vi "Read Waveform.vi"(8 "error in (no error)":errorcluster {"code" format="%.0x"}, 10 "Channel":string(combo)="Channel 1", 11 "VISA Resource Name":refnum<visa-resource-name>) -> (0 "error out":errorcluster {"code" format="%.0x"}, 1 "x increment":dbl caption="x Increment" format="%^.2e", 2 "initial x":dbl caption="Initial x" format="%^.2e", 3 "VISA Resource Name Out":refnum<visa-resource-name>, 4 "waveform array":dbl[](array[numeric]) caption="Waveform Array" format="%.2f", 5 "actual points":u32 caption="Actual Points")   [LabVIEW 2015, in "Agilent 546XX Series.lvlib"]
doc: "This VI initiates an acquisition on the channels that you enable with the ag546xx Configure Channel VI. It then waits for the acquisition to complete, and returns the waveform for the channel you specify. You call the ag546xx Fetch Waveform VI to obtain the waveforms for each of the remaining enabled channels without initiating another acquisition.\n\nNotes:\n\n(1) After this VI executes, each element in the Waveform Array is either a voltage or a value indicating that the oscilloscope could not sample a voltage."
uses:
  Agilent 546XX Series.lvlib
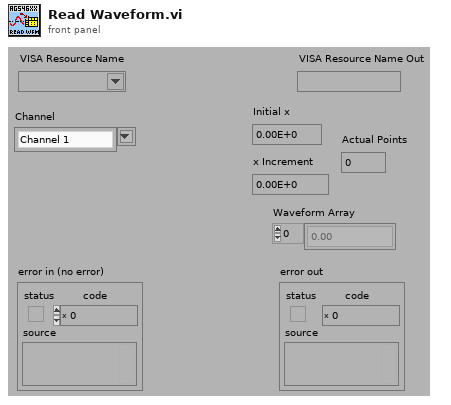
[diagram p1: front panel]
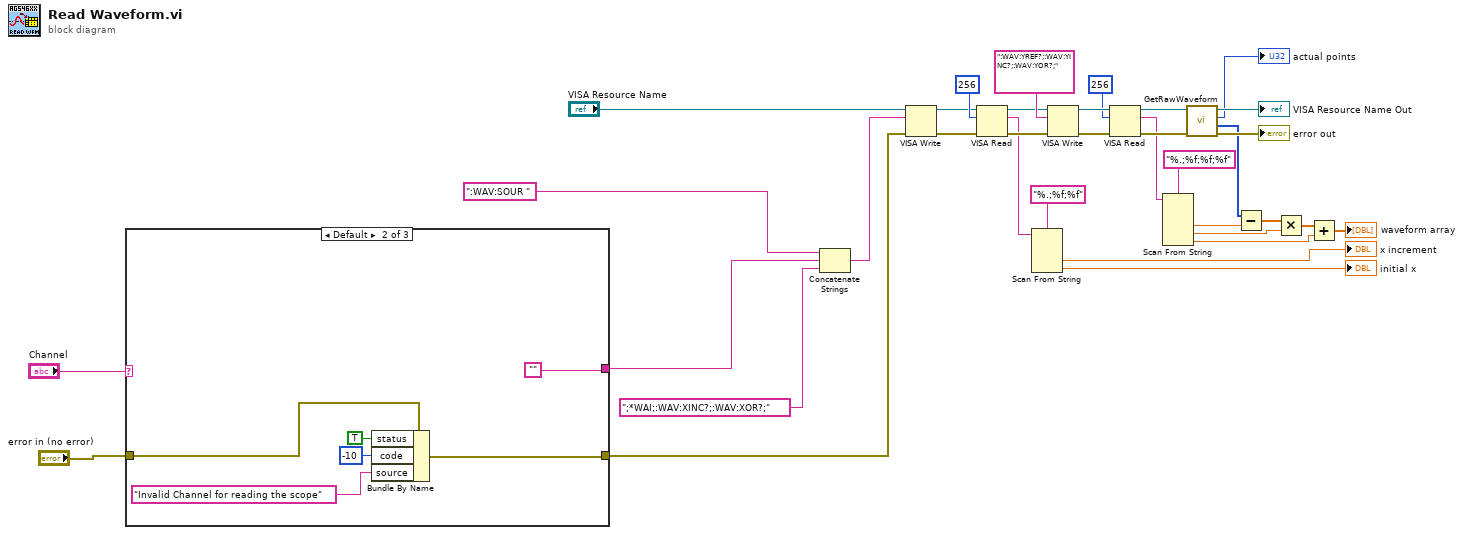
[diagram p0: block diagram]
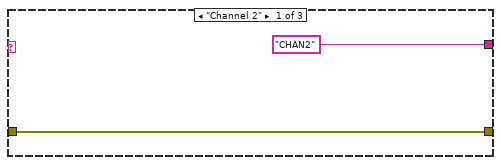
[diagram p2: hidden frame]
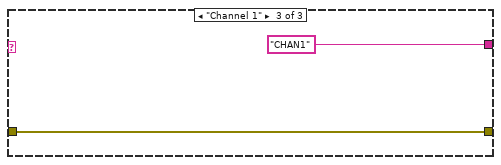
[diagram p3: hidden frame]
diagram:
  n1 = case shown="Default" "Channel" {
    tunnel: ["CHAN2" "" "CHAN1"] -> w6
    tunnel: "error in (no error)" -> [w36 w42 w44]
    tunnel: [w36 w38 w44] -> w1
    frame "Channel 2" {
    }
    frame Default {
      n2 = Bundle By Name(cluster=w42, "status"=TRUE, "code"=-10, "source"="Invalid Channel for reading the scope") -> (w38:errorcluster)
    }
    frame "Channel 1" {
    }
  }
  n3 = Concatenate Strings(":WAV:SOUR ", w6, ";*WAI;:WAV:XINC?;:WAV:XOR?;" ("string")) -> (w4:string)
  n4 = VISA Write(VISA resource name="VISA Resource Name", write buffer=w4, error in (no error)=w1) -> (VISA resource name out=w16:refnum<visa-resource-name>, error out=w15:errorcluster)  [unwired: 1 out]
  n5 = VISA Read(VISA resource name=w16, byte count=u32 256, error in (no error)=w15) -> (VISA resource name out=w14:refnum<visa-resource-name>, read buffer=w12:string, error out=w13:errorcluster)  [unwired: 1 out]
  n6 = Scan From String(format string="%.;%f;%f", input string=w12) -> (output 1=→"x increment":dbl, output 2=→"initial x":dbl)  [unwired: 4 in, 3 out]
  n7 = VISA Write(VISA resource name=w14, write buffer=":WAV:YREF?;:WAV:YINC?;:WAV:YOR?;", error in (no error)=w13) -> (VISA resource name out=w35:refnum<visa-resource-name>, error out=w34:errorcluster)  [unwired: 1 out]
  n8 = VISA Read(VISA resource name=w35, byte count=u32 256, error in (no error)=w34) -> (VISA resource name out=w33:refnum<visa-resource-name>, read buffer=w27:string, error out=w32:errorcluster)  [unwired: 1 out]
  n9 = Scan From String(format string="%.;%f;%f;%f", input string=w27) -> (output 1=w25:dbl, output 2=w23:dbl, output 3=w21:dbl)  [unwired: 5 in, 3 out]
  n10 = call "GetRawWaveform.vi"("error in"=w32, "VISA Resource Name"=w33) -> ("error out"=→"error out":errorcluster, "Waveform Array"=w19:u32[], "Number of Points"=→"actual points":u32, "VISA Resource Name Out"=→"VISA Resource Name Out":refnum<visa-resource-name>)  [unwired: 5 in, 1 out]
  n11 = Subtract(x=w19, y=w25) -> (x-y=w24:dbl[])
  n12 = Multiply(x=w24, y=w23) -> (x*y=w22:dbl[])
  n13 = Add(x=w22, y=w21) -> (x+y=→"waveform array":dbl[])
